vi "SetTimeout.vi"(8 "error in (no error)":errorcluster, 10 "Numeric":dbl, 11 "ThorLabsCsCamera in":refnum<class "ThorLabsCsCamera.lvclass">) -> (0 "error out":errorcluster, 3 "ThorLabsCsCamera out":refnum<class "ThorLabsCsCamera.lvclass">)   [LabVIEW 2020, in "ThorLabsCsCamera.lvclass"]
uses:
  ThorLabsCsCamera.lvclass
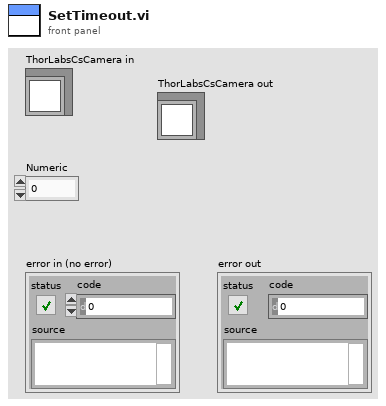
[diagram p1: front panel]
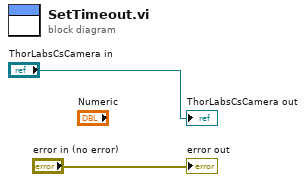
[diagram p0: block diagram]
diagram:
  "error out" <- "error in (no error)"
  "ThorLabsCsCamera out" <- "ThorLabsCsCamera in"
